vi "niFpgaRateLimiterTemplate.vi"(0 "input":fxp<+/-,16,16>, 1 "reset":bool, 5 "pos slew rate * dt":fxp<+/-,16,16>, 7 "neg slew rate * dt":fxp<+/-,16,16>) -> (4 "output":fxp<+/-,16,16>)   [LabVIEW 2017]
doc: "Specifies a maximum rate of change of a signal. The data type you wire to <B>input</B> determines the <B>output</B> data type."
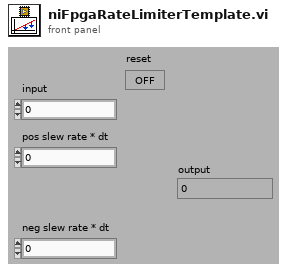
[diagram p1: front panel]
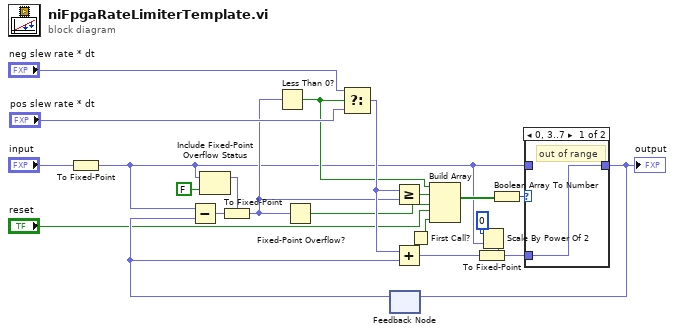
[diagram p0: block diagram]
diagram:
  n1 = To Fixed-Point(number="input") -> (fixed-point=w3:fxp<+/-,16,16>)  [unwired: 1 in]
  n2 = Include Fixed-Point Overflow Status(2:FALSE ("overflow"), 3:w3) -> (1:w9:fxp<+/-,16,16>)
  n3 = feedback #1() -> (w16:fxp<+/-,16,16>)  [unwired: 1 in]
  n4 = Subtract(x=w3, y=w16) -> (x-y=w15:fxp<+/-,17,17>)
  n5 = To Fixed-Point(fixed-point type=w9, number=w15) -> (fixed-point=w6:fxp<+/-,16,16>)
  n6 = Less Than 0?(x=w6) -> (x < 0?=w5:bool)
  n7 = Fixed-Point Overflow?(1:w6) -> (0:w7:bool)
  n8 = Select(t="neg slew rate * dt", s=w5, f="pos slew rate * dt") -> (s? t:f=w18:fxp<+/-,16,16>)
  n9 = Greater Or Equal?(x=w18, y=w6) -> (x >= y?=w22:bool)
  n10 = Add(x=w18, y=w16) -> (x+y=w17:fxp<+/-,17,17>)
  n11 = First Call?() -> (First Call?: T/F=w19:bool)
  n12 = Build Array(w5, w22, w7, "reset", w19) -> (w21:bool[])
  n13 = Scale By Power Of 2(n=0, x=w3) -> (x*2^n=w2:fxp<+/-,16,16>)
  n14 = To Fixed-Point(fixed-point type=w2, number=w17) -> (fixed-point=w8:fxp<+/-,16,16>)
  n15 = Boolean Array To Number(Boolean array=w21) -> (number=w20:u8)
  n16 = case shown="0, 3..7" w20 {
    tunnel: w8 -> [w23 _]
    tunnel: w3 -> [_ w24]
    tunnel: [w23 w24] -> w14
    frame 0, 3..7 {
      # "out of range"
    }
    frame 1, 2, Default {
      # "in range or \ninit"
    }
  }
  "output" <- w14
  n17 = feedback-in #1(w14) -> ()
